vi "Table Clear.vi"(8 "Error (In)":errorcluster, 11 "Table (In)":refnum<vi>) -> (0 "Error (Out)":errorcluster, 3 "Table (Out)":refnum<vi>)   [LabVIEW 2015]
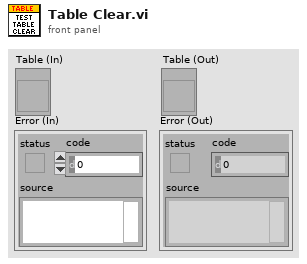
[diagram p1: front panel]
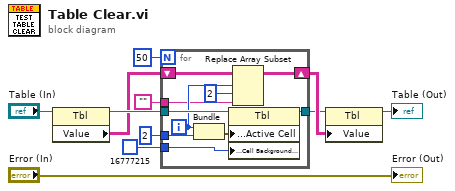
[diagram p0: block diagram]
diagram:
  n1 = property class="Tbl"(reference="Table (In)") -> (reference out=w7:refnum<vi>, "Value"=w4:string[][])  [unwired: 1 in, 1 out]
  n2 = for {
    N: 50 -> [_]
    tunnel: u32 16777215 -> [w20]
    tunnel: 2 -> [w19]
    tunnel: w7 -> [w18]
    tunnel: [w17] -> w1
    tunnel: "" -> [w14]
    shift-right: [w12] -> w3
    shift-left: w4 -> [w13]
    i -> [w16]
    n3 = Bundle(w16, w19) -> (w21:cluster{i32, i32})  [unwired: 1 in]
    n4 = property class="Tbl"(reference=w18, "Active Cell:Active Cell"=w21, "Active Cell:Cell Background Color"=w20) -> (reference out=w17:refnum<vi>)  [unwired: 1 in, 1 out]
    n5 = Replace Array Subset(array=w13, new element=w14, index (row)=w16, index (col)=2 ("disabled index (col)")) -> (w12:string[][])
  }
  n6 = property class="Tbl"(reference=w1, "Value"=w3) -> (reference out=→"Table (Out)":refnum<vi>)  [unwired: 1 in, 1 out]
  "Error (Out)" <- "Error (In)"
